vi "check_line_direction.vi"(7 "roi points in":i32[](array[numeric]), 8 "error in":errorcluster, 11 "final array in":u16[][](array[numeric])) -> (0 "error out":errorcluster, 3 "Array":u16[][](array[numeric]))   [LabVIEW 2010, in "TrajectoryMH100122AODRAPS.lvclass"]
uses:
  TrajectoryMH100122AODRAPS.lvclass
  <vilib>/Analysis/NI_AALPro.lvlib
  <vilib>/gmath/NI_Gmath.lvlib
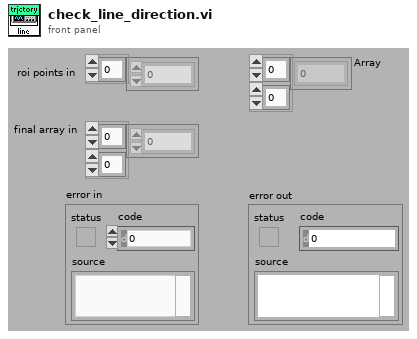
[diagram p1: front panel]
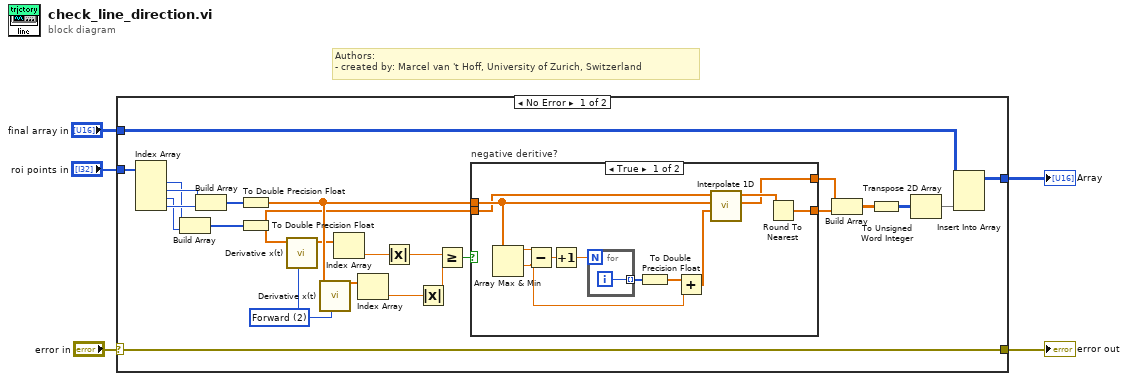
[diagram p0: block diagram]
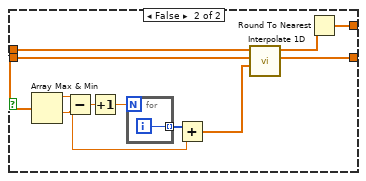
[diagram p2: hidden frame]
diagram:
  # "Authors: \n- created by: Marcel van 't Hoff, University of Zurich, Switzerland"
  n1 = case shown="No Error" "error in" {
    selector: "error in" -> [w6 w56]
    tunnel: [w14 _] -> w5
    tunnel: "final array in" -> [w12 _]
    tunnel: "roi points in" -> [w7 _]
    tunnel: [w6 w56] -> w1
    frame No Error {
      w23 = u16 2 items=["2nd Order Central", "4th Order Central", "Forward", "Backward"] ("method")
      n2 = Index Array(array=w7) -> (element #1=w8:i32, element #2=w10:i32, element #3=w9:i32, element #4=w11:i32)  [unwired: 4 in]
      n3 = Build Array(w8, w9) -> (w22:i32[])
      n4 = Build Array(w10, w11) -> (w15:i32[])
      n5 = To Double Precision Float(number=w15) -> (double precision float=w30:dbl[])
      n6 = To Double Precision Float(number=w22) -> (double precision float=w29:dbl[])
      n7 = call <vilib>:"Derivative x(t).vi"("method"=w23, "X"=w29) -> ("dX/dt"=w24:dbl[])  [unwired: 8 in, 1 out]
      n8 = call <vilib>:"Derivative x(t).vi"("method"=w23, "X"=w30) -> ("dX/dt"=w16:dbl[])  [unwired: 8 in, 1 out]
      n9 = Index Array(array=w24) -> (element=w25:dbl)  [unwired: 1 in]
      n10 = Index Array(array=w16) -> (element=w26:dbl)  [unwired: 1 in]
      n11 = Absolute Value(x=w25) -> (abs(x)=w27:dbl)
      n12 = Absolute Value(x=w26) -> (abs(x)=w28:dbl)
      n13 = Greater Or Equal?(x=w27, y=w28) -> (x >= y?=w17:bool)
      n14 = case "negative deritive?" shown="True" w17 {
        tunnel: [w32 w53] -> w19
        tunnel: [w33 w52] -> w18
        tunnel: w29 -> [w34 w45]
        tunnel: w30 -> [w35 w51]
        frame True {
          n15 = Array Max & Min(array=w35) -> (max value=w37:dbl, min value=w39:dbl)  [unwired: 2 out]
          n16 = Subtract(x=w37, y=w39) -> (x-y=w38:dbl)
          n17 = Increment(x=w38) -> (x+1=w41:dbl)
          n18 = for {
            N: w41 -> [_]
            tunnel: [w43] -> w40 mode=indexing
            i -> [w43]
          }
          n19 = To Double Precision Float(number=w40) -> (double precision float=w31:dbl[])
          n20 = Add(x=w31, y=w39) -> (x+y=w36:dbl[])
          n21 = call <vilib>:"Interpolate 1D.vi"("xi"=w36, "X"=w35, "Y"=w34) -> ("xi used"=w33:dbl[], "yi"=w42:dbl[])  [unwired: 6 in, 1 out]
          n22 = Round To Nearest(number=w42) -> (nearest integer value=w32:dbl[])
        }
        frame False {
          n23 = Array Max & Min(array=w45) -> (max value=w46:dbl, min value=w48:dbl)  [unwired: 2 out]
          n24 = Subtract(x=w46, y=w48) -> (x-y=w47:dbl)
          n25 = Increment(x=w47) -> (x+1=w50:dbl)
          n26 = for {
            N: w50 -> [_]
            tunnel: [w55] -> w49 mode=indexing
            i -> [w55]
          }
          n27 = Add(x=w49, y=w48) -> (x+y=w44:dbl[])
          n28 = call <vilib>:"Interpolate 1D.vi"("xi"=w44, "X"=w45, "Y"=w51) -> ("xi used"=w53:dbl[], "yi"=w54:dbl[])  [unwired: 6 in, 1 out]
          n29 = Round To Nearest(number=w54) -> (nearest integer value=w52:dbl[])
        }
      }
      n30 = Build Array(w18, w19) -> (w20:dbl[][])
      n31 = To Unsigned Word Integer(number=w20) -> (unsigned 16bit integer=w21:u16[][])
      n32 = Transpose 2D Array(2D array=w21) -> (transposed array=w13:u16[][])
      n33 = Insert Into Array(array=w12, new element=w13) -> (w14:u16[][])  [unwired: 2 in]
    }
    frame Error {
    }
  }
  "Array" <- w5
  "error out" <- w1
